vi "GenExcitationString.vi"(11 "Pulse Sequence":T1(array[cluster])) -> (3 "Emission Filter String":string)   [LabVIEW 2010, in "Settings.lvclass"]
uses:
  Settings.lvclass
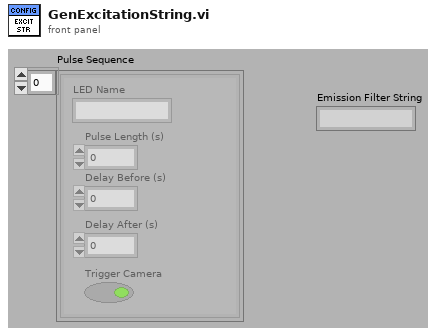
[diagram p1: front panel]
types:
  T1 = cluster{"LED Name":string, "Pulse Length (s)":dbl, "Delay Before (s)":dbl, "Delay After (s)":dbl, "Trigger Camera":bool}[]
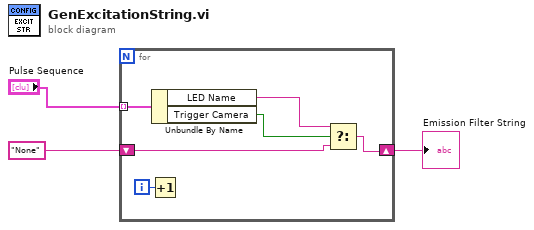
[diagram p0: block diagram]
diagram:
  n1 = for {
    tunnel: "Pulse Sequence" -> [w8] mode=indexing
    shift-right: [w6] -> w1
    shift-left: "None" ("Emission Filter String") -> [w7]
    i -> [w9]
    n2 = Increment(x=w9) -> ()  [unwired: 1 out]
    n3 = Unbundle By Name(w8) -> ("LED Name"=w4:string, "Trigger Camera"=w5:bool)
    n4 = Select(t=w4, s=w5, f=w7) -> (s? t:f=w6:string)
  }
  "Emission Filter String" <- w1
